vi "XY Graph Get Multiplot Action Message.vi"(8 "error in (no error)":errorcluster, 9 "Graph Action":string, 10 "Graph Caption":string, 11 "Plot Names":string[](array[string])) -> (0 "Error Out":errorcluster, 3 "Multiplot Message":string)   [LabVIEW 2021, in "XY Graph Add-Ons.lvlib"]
uses:
  XY Graph Add-Ons.lvlib
  Strings/Strings.lvlib
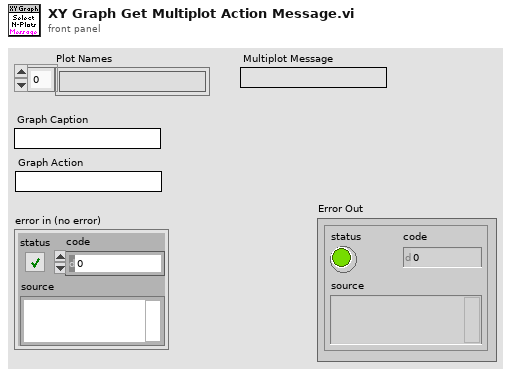
[diagram p1: front panel]
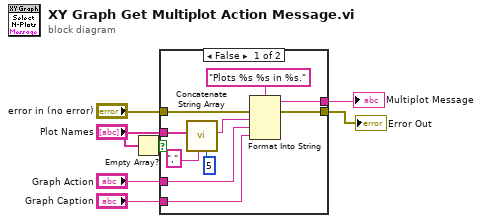
[diagram p0: block diagram]
diagram:
  n1 = Empty Array?(array="Plot Names") -> (empty?=w3:bool)
  n2 = case shown="False" w3 {
    tunnel: "Plot Names" -> [w14 _]
    tunnel: "error in (no error)" -> [w13 w18]
    tunnel: "Graph Caption" -> [w12 _]
    tunnel: [w10 _] -> w7
    tunnel: [w9 w18] -> w1
    tunnel: "Graph Action" -> [w8 _]
    frame False {
      n3 = call "Concatenate String Array.vi"("Max Number of Elements (None: -1)"=5 ("Max Number of Elements (None: 1)"), "Separator (TAB)"=",", "String Array"=w14) -> ("Formatted String"=w17:string)  [unwired: 8 in]
      n4 = Format Into String(format string="Plots %s %s in %s.", error in=w13, w17, w8, w12) -> (resulting string=w10:string, error out=w9:errorcluster)  [unwired: 1 in]
    }
    frame True {
    }
  }
  "Multiplot Message" <- w7
  "Error Out" <- w1
